vi "Enabling rec buttons behaviour.vi"(9 "Live img":bool, 11 "New Value":bool) -> ()   [LabVIEW 2013]
uses:
  Typedefs/Read Write Enum.ctl
  Global Variables/gl_UI Ctrl Refs.vi
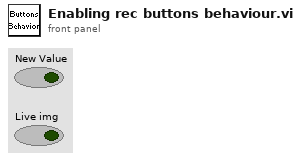
[diagram p1: front panel]
types:
  T1 = typedef "Read Write Enum.ctl" = enum16{"Read", "Write"}
  T2 = typedef "UI ctrl refs cluster.ctl" = cluster{"Top level VI path":path, "Top level VI ref":refnum<vi>, "User menu ref":refnum<k9>, "Sub Panel control":refnum<vi>, "Imaging Param Tab":refnum<vi>, "Occurrence-Start drivers":refnum<k4>, "Occurrence-Speed logging initialised":refnum<k4>, "Occurrence-XYZ stage initialised":refnum<k4>, "Exit button":refnum<vi>, "Status ind":refnum<vi>, "Return to Origin":refnum<vi>, "Speed Logging":refnum<vi>, "Time Lapse":refnum<vi>, "Live Imaging":refnum<vi>, "AOL Z Stack":refnum<vi>, "Motor Z Stack":refnum<vi>, "Funct Acq button":refnum<vi>, "Hard Shutter":refnum<vi>, "Virtual Shutter":refnum<vi>, "Laser Power":refnum<vi>, "AOL Mode":refnum<vi>, "Frame Size":refnum<vi>, "Field of View":refnum<vi>, "Dwell Time":refnum<vi>, "Zoom":refnum<vi>, "AOL Z":refnum<vi>, "Objective":refnum<vi>, "Axis":refnum<vi>, "Paths & Names":refnum<vi>, "Experiment folder path (ind.)":refnum<vi>, "Last State (Ind.)":refnum<vi>, "Laser wavelength ind (nm)":refnum<vi>, "Averages":refnum<vi>, "Angle (degrees)":refnum<vi>, "X centre":refnum<vi>, "Y centre":refnum<vi>, "Plane Mode":refnum<vi>, "# Planes":refnum<vi>, "Z Start":refnum<vi>, "Z Stop":refnum<vi>, "Z Step":refnum<vi>, "PMT 1":refnum<vi>, "PMT 2":refnum<vi>, "Stage XYZ Position":refnum<vi>, "Pockels@Z Start":refnum<vi>, "Pockels@Z Stop":refnum<vi>, "Obtain Z Start":refnum<vi>, "Obtain Z Stop":refnum<vi>, "Live stim.trig.period":refnum<vi>, "Live stim.trig.enable":refnum<vi>, "Funct. Acq. Pockels Modulation":refnum<vi>, "Enable Video Recording":refnum<vi>, "Video Record-Live Imaging":refnum<vi>, "Video Record-Funct acq":refnum<vi>, "AOL Z-stack Chirps Ready (ind)":refnum<vi>, "Center freq ind (nm)":refnum<vi>, "Logging queue (ind)":refnum<vi>, "Back aperture power (ind.)":refnum<vi>, "Power after objective (ind.)":refnum<vi>, "Switch user":refnum<vi>}
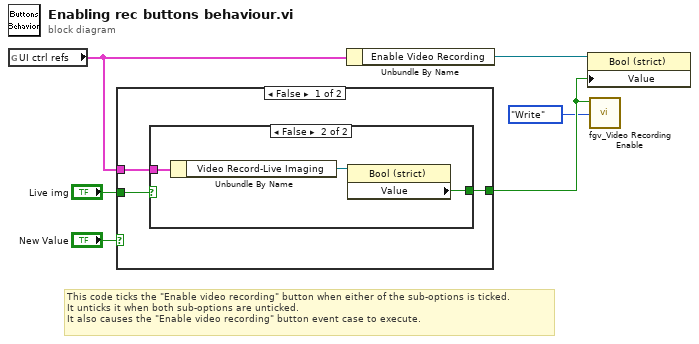
[diagram p0: block diagram]
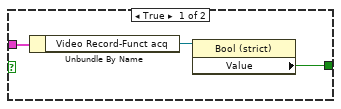
[diagram p2: hidden frame]
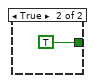
[diagram p3: hidden frame]
diagram:
  # "This code ticks the \"Enable video recording\" button when either of the sub-options is ticked.\nIt unticks it when both sub-options are unticked.\nIt also causes the \"Enable video recording\" button event case to execute."
  n1 = global read "gl_UI Ctrl Refs.vi" "UI ctrl refs"() -> (w3:T2)
  n2 = case shown="False" "New Value" {
    tunnel: w3 -> [w8 _]
    tunnel: "Live img" -> [w9 _]
    tunnel: [w7 TRUE ("Value (Signaling)")] -> w2
    frame False {
      n3 = case shown="False" w9 {
        tunnel: w8 -> [w11 w14]
        tunnel: [w10 w13] -> w7
        frame True {
          n4 = Unbundle By Name(w11) -> ("Video Record-Funct acq"=w12:refnum<vi>)
          n5 = property class="Bool (strict)"(reference=w12) -> ("Value"=w10:bool)  [unwired: 1 in, 2 out]
        }
        frame False {
          n6 = Unbundle By Name(w14) -> ("Video Record-Live Imaging"=w15:refnum<vi>)
          n7 = property class="Bool (strict)"(reference=w15) -> ("Value"=w13:bool)  [unwired: 1 in, 2 out]
        }
      }
    }
    frame True {
    }
  }
  n8 = Unbundle By Name(w3) -> ("Enable Video Recording"=w4:refnum<vi>)
  n9 = property class="Bool (strict)"(reference=w4, "Value"=w2) -> ()  [unwired: 1 in, 2 out]
  n10 = call "fgv_Video Recording Enable.vi"("Function"=Read_Write_Enum."Write", "Video Recording Enabled"=w2) -> ()  [unwired: 9 in, 1 out]
